vi "Release.vi"(8 "error in (no error)":errorcluster, 11 "QMenu Class in":refnum<class "QMenu Class.lvclass">) -> (0 "error out":errorcluster)   [LabVIEW 2020, in "QTab.lvlib" / "QMenu Class.lvclass"]
uses:
  QMenu Class.lvclass
  QMenu Class.lvclass/QMenu Class.ctl
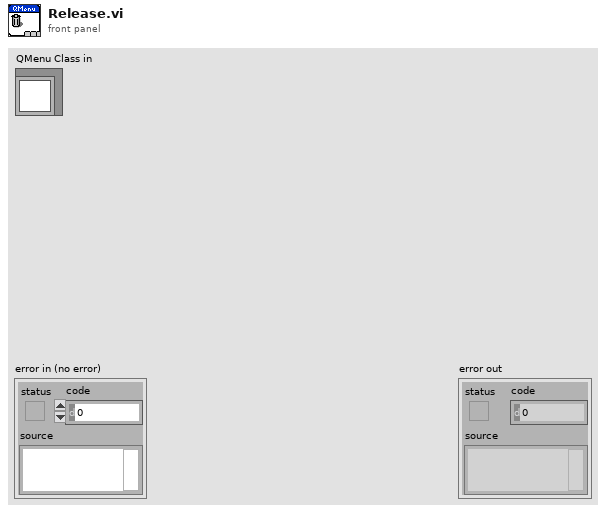
[diagram p1: front panel]
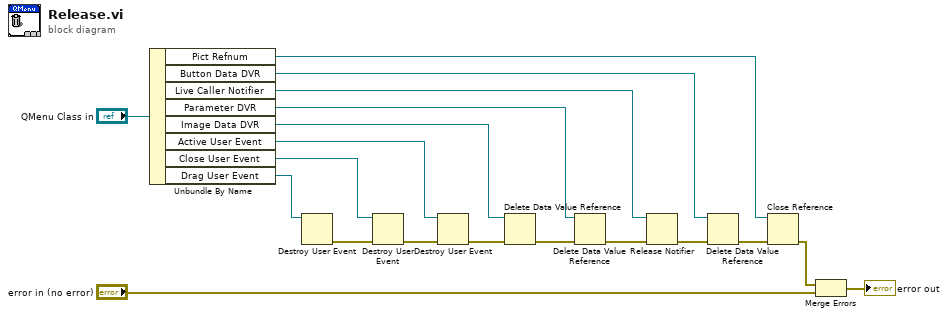
[diagram p0: block diagram]
diagram:
  n1 = Unbundle By Name("QMenu Class in") -> ("Pict Refnum"=w18:refnum<vi>, "Button Data DVR"=w13:refnum<data-value>, "Live Caller Notifier"=w11:refnum<notifier>, "Parameter DVR"=w2:refnum<data-value>, "Image Data DVR"=w10:refnum<data-value>, "Active User Event"=w8:refnum<user-event>, "Close User Event"=w6:refnum<user-event>, "Drag User Event"=w4:refnum<user-event>)
  n2 = Destroy User Event(user event=w4) -> (error out=w5:errorcluster)  [unwired: 1 in]
  n3 = Destroy User Event(user event=w6, error in=w5) -> (error out=w7:errorcluster)
  n4 = Destroy User Event(user event=w8, error in=w7) -> (error out=w9:errorcluster)
  n5 = Delete Data Value Reference(data value reference=w10, error in=w9) -> (error out=w3:errorcluster)  [unwired: 1 out]
  n6 = Delete Data Value Reference(data value reference=w2, error in=w3) -> (error out=w1:errorcluster)  [unwired: 1 out]
  n7 = Release Notifier(notifier=w11, error in (no error)=w1) -> (error out=w12:errorcluster)  [unwired: 1 in, 2 out]
  n8 = Delete Data Value Reference(data value reference=w13, error in=w12) -> (error out=w14:errorcluster)  [unwired: 1 out]
  n9 = Close Reference(reference=w18, error in (no error)=w14) -> (error out=w17:errorcluster)
  n10 = Merge Errors(w17, "error in (no error)") -> (→"error out":errorcluster)
